vi "Handle Error.vi"(8 "error in (no error)":errorcluster, 11 "IModel in":refnum<class "IModel.lvclass">) -> (0 "error out":errorcluster, 2 "stop actor?":bool=TRUE, 3 "IModel out":refnum<class "IModel.lvclass">)   [LabVIEW 2020, in "IModel.lvlib" / "IModel.lvclass"]
uses:
  <vilib>/gpm_packages/@cs/mva-core/Source/IModel/IModel/IModel.lvclass
  C:/Program Files/National Instruments/LabVIEW 2020/vi.lib/ActorFramework/Actor/Actor.lvclass
  <vilib>/ActorFramework/Actor/Actor.lvclass/Actor.ctl
  <vilib>/ActorFramework/Message Enqueuer/Message Enqueuer.lvclass/Message Enqueuer.ctl
  <vilib>/ActorFramework/Stop Msg/Stop Msg.lvclass/Stop Msg.ctl
  <vilib>/ActorFramework/Message Enqueuer/Enqueue Critical.vi
  <vilib>/ActorFramework/Message Enqueuer/Init from Existing Queue.vi
  <vilib>/ActorFramework/Stop Msg/Stop Msg.lvclass
  C:/Program Files/National Instruments/LabVIEW 2020/vi.lib/ActorFramework/Message/Message.lvclass
  <vilib>/ActorFramework/Message Priority Queue/Priority Enqueue.vi
  <vilib>/gpm_packages/@cs/mva-core/Source/IObserver/IObserver/IObserver.lvclass
  <vilib>/ActorFramework/Message Enqueuer/Message Enqueuer.lvclass
  <vilib>/ActorFramework/Actor/Actor.lvclass
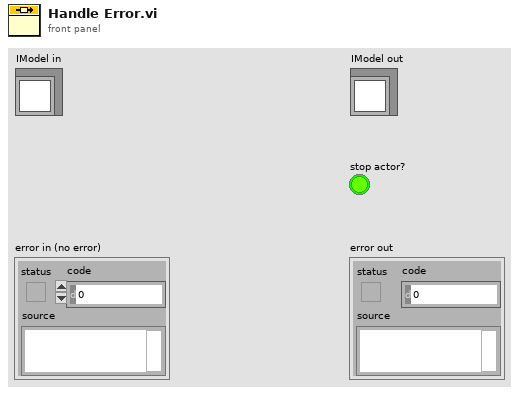
[diagram p1: front panel]
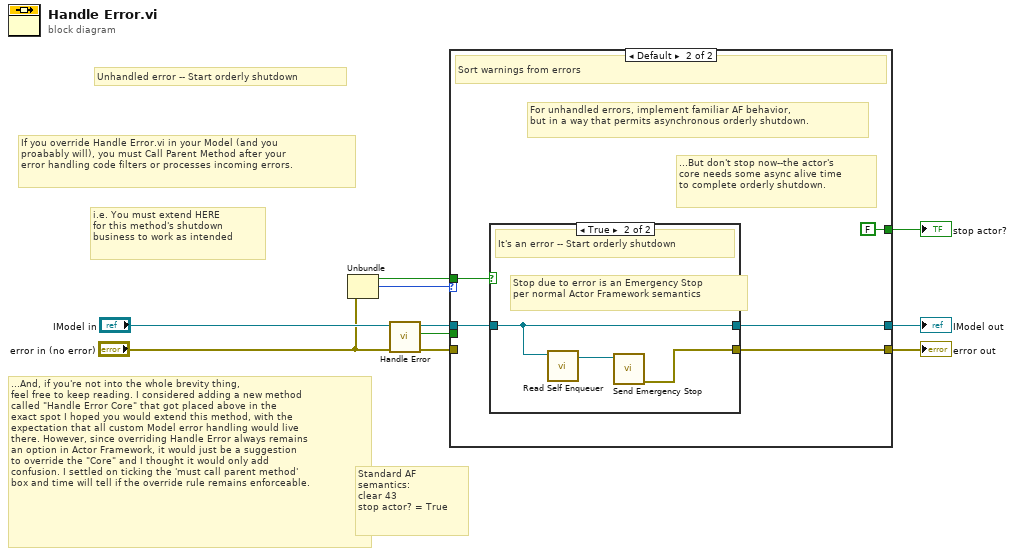
[diagram p0: block diagram]
diagram:
  # "Standard AF\nsemantics:\nclear 43\nstop actor? = True"
  # "Unhandled error -- Start orderly shutdown"
  # "...And, if you're not into the whole brevity thing,\nfeel free to keep reading. I considered adding a new method\ncalled \"Handle Error Core\" that got placed above in the\nexact spot I hoped you would extend this method, with the\nexpectation that all custom Model error handling would live\nthere. However, since overriding Handle Error always remains\nan option in Actor Framework, it would just be a suggestion\nto override the \"Core\" and I thought it would only add\nconfusion. I settled on ticking the 'must call parent method'\nbox and time will tell if the override rule remains enforceable."
  # "i.e. You must extend HERE\nfor this method's shutdown\nbusiness to work as intended"
  # "If you override Handle Error.vi in your Model (and you\nproabably will), you must Call Parent Method after your\nerror handling code filters or processes incoming errors."
  n1 = Unbundle("error in (no error)") -> ("status"=w1:bool, "code"=w7:i32)  [unwired: 1 out]
  n2 = call-parent "Handle Error.vi"("error in (no error)"="error in (no error)", "IObserver in"="IModel in") -> ("error out"=w3:errorcluster, "stop actor?"=w2:bool, "IObserver out"=w5:refnum<class "IModel.lvclass">)  [unwired: 7 in]
  n3 = case shown="Default" w7 {
    tunnel: w3 -> [w13 _]
    tunnel: w5 -> [w12 w16]
    tunnel: [w12 w14] -> w9
    tunnel: [w13 w18] -> w8
    tunnel: [w11 FALSE ("stop actor?")] -> w6
    tunnel: w2 -> [w11 _]
    tunnel: w1 -> [_ w15]
    frame 43, 1608 {
      # "43 = Normal Actor shutdown\n1608 = Emergency Actor shutdown\n\nWhen a stop msg gets invoked via Do.vi (and then gets\nhere) it is actually time to stop--so let it through!\n\nIf you returned a 43 or 1608 error directly from a method\nto force an immediate stop, this Actor believes you and\nstops without performing orderly shutdown. Do that at\nyour own risk and, ideally, only with a Model that does\nnot expect to collect any nested Models (You might also\nconsider using the method 'Send Immediate Stop'.)"
      # "Handle final Actor shutdown codes"
    }
    frame Default {
      # "For unhandled errors, implement familiar AF behavior,\nbut in a way that permits asynchronous orderly shutdown."
      # "...But don't stop now--the actor's\ncore needs some async alive time\nto complete orderly shutdown."
      # "Sort warnings from errors"
      n4 = case shown="True" w15 {
        tunnel: [_ w21] -> w18
        tunnel: w16 -> [w19 w20]
        tunnel: [w19 w20] -> w14
        frame False {
          # "Error was cleared or it's just a warning"
        }
        frame True {
          # "Stop due to error is an Emergency Stop\nper normal Actor Framework semantics"
          # "It's an error -- Start orderly shutdown"
          n5 = call <vilib>:"Read Self Enqueuer.vi"("Actor"=w20) -> ("Self Enqueuer"=w22:refnum<class "Message Enqueuer.lvclass">)  [unwired: 10 in]
          n6 = call <vilib>:"Send Emergency Stop.vi"("Message Enqueuer"=w22) -> ("error out"=w21:errorcluster)  [unwired: 10 in]
        }
      }
    }
  }
  "IModel out" <- w9
  "error out" <- w8
  "stop actor?" <- w6
